vi "Shutdown.vi"(8 "error in (no error)":errorcluster, 11 "Engine in":refnum<class "Engine.lvclass">) -> (0 "error out":errorcluster, 3 "Engine out":refnum<class "Engine.lvclass">)   [LabVIEW 2023, in "Engine.lvlib" / "Engine.lvclass"]
doc: "<b>Shutdown</b>\nThis routine is implemented in the stop actor override -> as a result, it is not necessary to call shutdown anywhere else, and any methods that need to be called prior to stop actor core can be implemented here.\n\n<b>Engine</b> - No methods implemented at the engine level"
uses:
  Library/Engine.lvclass
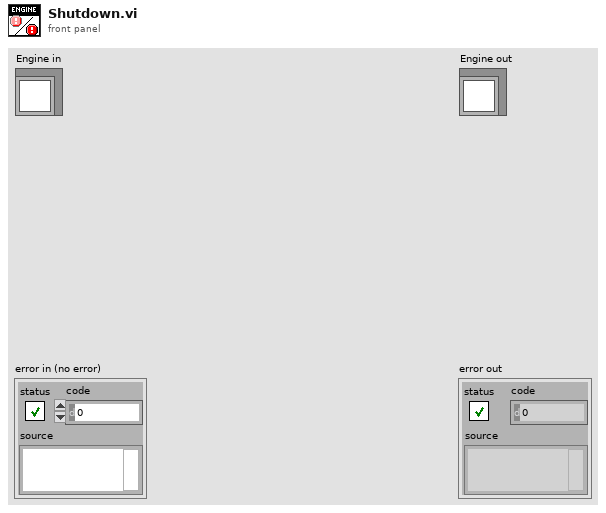
[diagram p1: front panel]
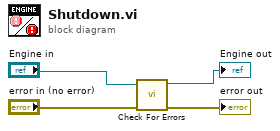
[diagram p0: block diagram]
diagram:
  n1 = call "Check For Errors.vi"("error in"="error in (no error)", "Engine in"="Engine in") -> ("error out"=→"error out":errorcluster, "Engine out"=→"Engine out":refnum<class "Engine.lvclass">)  [unwired: 8 in]
